vi "ODE formula string function.vi"(2 "function parameters":variant, 3 "time":dbl, 4 "X":dbl[](array[numeric])) -> (0 "error out":errorcluster, 1 "F(X,time)":dbl[](array[numeric]))   [LabVIEW 2018, in "NI_Gmath.lvlib"]
uses:
  NI_Gmath.lvlib
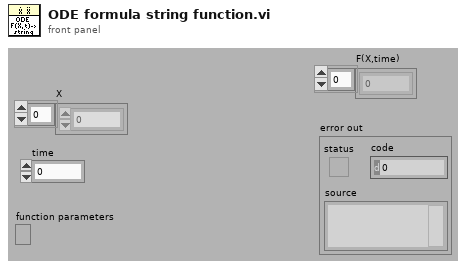
[diagram p1: front panel]
types:
  T1 = cluster{"F(X,t)":string[], "X":string[], "time":string}
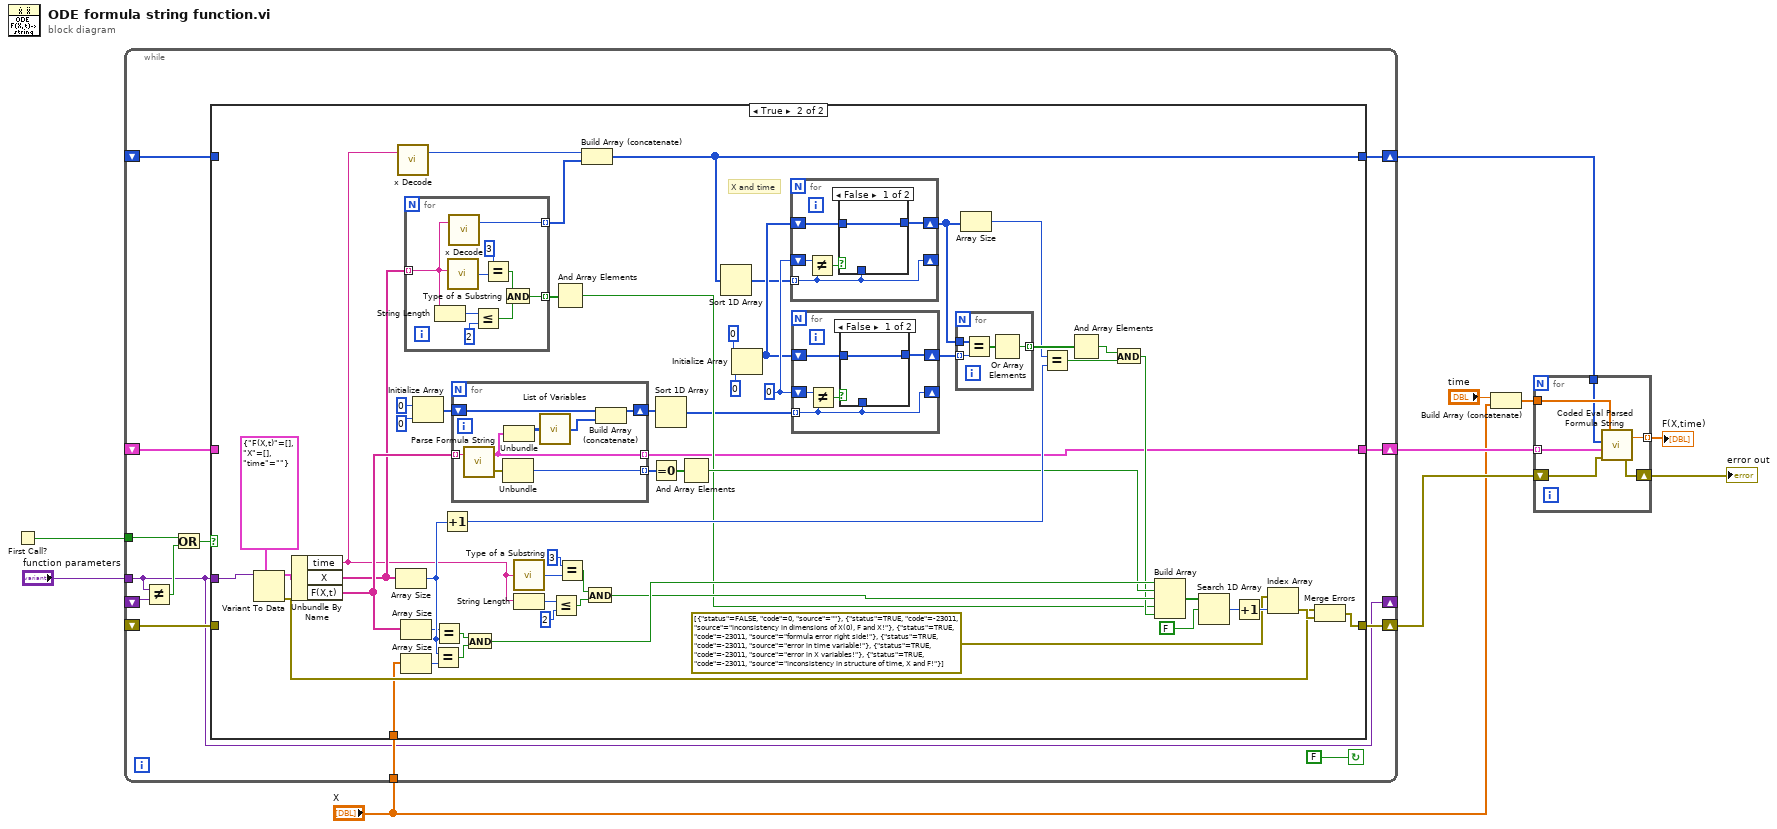
[diagram p0: block diagram]
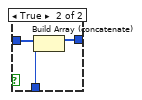
[diagram p3: hidden frame]
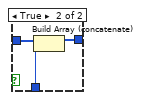
[diagram p4: hidden frame]
diagram:
  n1 = First Call?() -> (First Call?: T/F=w10:bool)
  n2 = while {
    tunnel: w10 -> [w13]
    tunnel: "function parameters" -> [w11]
    shift-right: [w20] -> w4
    shift-left: _ -> [w19]
    shift-right: [w22] -> w2
    shift-left: _ -> [w21]
    shift-right: [w18] -> w3
    shift-left: _ -> [w17]
    tunnel: "X" -> [w16]
    shift-right: [w11] -> _
    shift-left: _ -> [w15]
    stop <- FALSE continue-if-true
    n3 = Not Equal?(x=w11, y=w15) -> (x != y?=w14:bool)
    n4 = Or(x=w13, y=w14) -> (x .or. y?=w12:bool)
    n5 = case shown="True" w12 {
      tunnel: w11 -> [_ w81]
      tunnel: [w26 w44] -> w22
      tunnel: w21 -> [w26 _]
      tunnel: [w25 w31] -> w20
      tunnel: w19 -> [w25 _]
      tunnel: [w24 w40] -> w18
      tunnel: w17 -> [w24 _]
      tunnel: w16 -> [_ w27]
      frame False {
      }
      frame True {
        w37 = 0
        # "X and time"
        n6 = Variant To Data(type=T1 {"F(X,t)"=[], "X"=[], "time"=""}, Variant=w81) -> (data=w59:T1, error out=w45:errorcluster)  [unwired: 1 in]
        n7 = Unbundle By Name(w59) -> ("time"=w43:string, "X"=w57:string[], "F(X,t)"=w58:string[])
        n8 = Array Size(array=w57) -> (size(s)=w77:i32)
        n9 = call "x Decode.vi"("x string"=w43) -> ("number"=w41:i32)  [unwired: 1 in, 1 out]
        n10 = Array Size(array=w58) -> (size(s)=w62:i32)
        n11 = Array Size(array=w27) -> (size(s)=w63:i32)
        n12 = for {
          tunnel: w57 -> [w105] mode=indexing
          tunnel: [w106] -> w72 mode=indexing
          tunnel: [w104] -> w42 mode=indexing
          n13 = String Length(string=w105) -> (length=w107:i32)
          n14 = call "Type of a Substring.VI"("item"=w105) -> ("type"=w109:i32)
          n15 = call "x Decode.vi"("x string"=w105) -> ("number"=w104:i32)  [unwired: 1 in, 1 out]
          n16 = Less Or Equal?(x=w107, y=2) -> (x <= y?=w111:bool)
          n17 = Equal?(x=3, y=w109) -> (x = y?=w112:bool)
          n18 = And(x=w112, y=w111) -> (x .and. y?=w106:bool)
        }
        n19 = Initialize Array(0, 0) -> (w75:i32[])
        n20 = Equal?(x=w77, y=w63) -> (x = y?=w64:bool)
        n21 = Equal?(x=w62, y=w77) -> (x = y?=w65:bool)
        n22 = Increment(x=w77) -> (x+1=w78:i32)
        n23 = for {
          tunnel: [w115] -> w61 mode=indexing
          tunnel: w58 -> [w120] mode=indexing
          shift-right: [w118] -> w76
          shift-left: w75 -> [w119]
          tunnel: [w113] -> w40 mode=indexing
          n24 = call "Parse Formula String.vi"("formula"=w120) -> ("error out"=w116:errorcluster, "Parsed Formula"=w113:cluster{"Table":i32[][], "Y Values":dbl[]})  [unwired: 1 in]
          n25 = Unbundle(w116) -> ("code"=w115:i32)  [unwired: 2 out]
          n26 = Unbundle(w113) -> ("Table"=w114:i32[][])  [unwired: 1 out]
          n27 = call "List of Variables.vi"("Table"=w114) -> ("List of variables"=w117:i32[])
          n28 = Build Array (concatenate)(w119, w117) -> (w118:i32[])
        }
        n29 = And(x=w65, y=w64) -> (x .and. y?=w56:bool)
        n30 = call "Type of a Substring.VI"("item"=w43) -> ("type"=w68:i32)
        n31 = String Length(string=w43) -> (length=w66:i32)
        n32 = Less Or Equal?(x=w66, y=2) -> (x <= y?=w70:bool)
        n33 = And Array Elements(Boolean array=w72) -> (logical AND=w52:bool)
        n34 = Equal?(x=3, y=w68) -> (x = y?=w71:bool)
        n35 = Build Array (concatenate)(w41, w42) -> (w31:i32[])
        n36 = And(x=w71, y=w70) -> (x .and. y?=w54:bool)
        n37 = Equal To 0?(x=w61) -> (x = 0?=w60:bool[])
        n38 = Sort 1D Array(array=w76) -> (sorted array=w30:i32[])
        n39 = And Array Elements(Boolean array=w60) -> (logical AND=w55:bool)
        n40 = Sort 1D Array(array=w31) -> (sorted array=w35:i32[])
        n41 = Initialize Array(0, 0) -> (w36:i32[])
        n42 = for {
          shift-right: [w92] -> w33
          shift-left: w36 -> [w93]
          shift-right: [w91] -> _
          shift-left: w37 -> [w95]
          tunnel: w35 -> [w91] mode=indexing
          n43 = Not Equal?(x=w95, y=w91) -> (x != y?=w94:bool)
          n44 = case shown="False" w94 {
            tunnel: w93 -> [w96 w99]
            tunnel: [w96 w98] -> w92
            tunnel: w91 -> [_ w97]
            frame False {
            }
            frame True {
              n45 = Build Array (concatenate)(w99, w97) -> (w98:i32[])
            }
          }
        }
        n46 = for {
          shift-right: [w83] -> w34
          shift-left: w36 -> [w84]
          shift-right: [w82] -> _
          shift-left: w37 -> [w86]
          tunnel: w30 -> [w82] mode=indexing
          n47 = Not Equal?(x=w86, y=w82) -> (x != y?=w85:bool)
          n48 = case shown="False" w85 {
            tunnel: w84 -> [w87 w90]
            tunnel: [w87 w89] -> w83
            tunnel: w82 -> [_ w88]
            frame False {
            }
            frame True {
              n49 = Build Array (concatenate)(w90, w88) -> (w89:i32[])
            }
          }
        }
        n50 = for {
          tunnel: w34 -> [w103] mode=indexing
          tunnel: w33 -> [w102]
          tunnel: [w100] -> w32 mode=indexing
          n51 = Equal?(x=w102, y=w103) -> (x = y?=w101:bool[])
          n52 = Or Array Elements(Boolean array=w101) -> (logical OR=w100:bool)
        }
        n53 = Array Size(array=w33) -> (size(s)=w29:i32)
        n54 = Equal?(x=w29, y=w78) -> (x = y?=w79:bool)
        n55 = And Array Elements(Boolean array=w32) -> (logical AND=w28:bool)
        n56 = And(x=w28, y=w79) -> (x .and. y?=w53:bool)
        n57 = Build Array(w56, w55, w54, w52, w53) -> (w51:bool[])
        n58 = Search 1D Array(1D array=w51, element=FALSE) -> (index of element=w49:i32)  [unwired: 1 in]
        n59 = Increment(x=w49) -> (x+1=w48:i32)
        n60 = Index Array(array=errorcluster[] [{"status"=FALSE, "code"=0, "source"=""}, {"status"=TRUE, "code"=-23011, "source"="inconsistency in dimensions of X(0), F and X!"}, {"status"=TRUE, "code"=-23011, "source"="formula error right side!"}, {"status"=TRUE, "code"=-23011, "source"="error in time variable!"}, {"status"=TRUE, "code"=-23011, "source"="error in X variables!"}, {"status"=TRUE, "code"=-23011, "source"="inconsistency in structure of time, X and F!"}], index=w48) -> (element=w47:errorcluster)
        n61 = Merge Errors(w45, w47) -> (w44:errorcluster)
      }
    }
  }
  n62 = Build Array (concatenate)("time", "X") -> (w7:dbl[])
  n63 = for {
    tunnel: w4 -> [w124]
    tunnel: w7 -> [w125]
    tunnel: [w126] -> w6 mode=indexing
    shift-right: [w122] -> w5
    shift-left: w2 -> [w123]
    tunnel: w3 -> [w121] mode=indexing
    n64 = call "Coded Eval Parsed Formula String.vi"("error in (no error)"=w123, "Parsed Formula"=w121, "Variables"=w124, "X Values"=w125) -> ("error out"=w122:errorcluster, "y value"=w126:dbl)
  }
  "error out" <- w5
  "F(X,time)" <- w6
